vi "ArduinoSerial.vi"() -> ()   [LabVIEW 2014]
uses:
  <vilib>/Instr/_visa.llb/VISA Configure Serial Port (Instr).vi
panel:
  out "XY Graph":cluster{dbl[], dbl[]}(graph)
  out "Y":dbl
  out "X":dbl
  in  "VISA resource name":refnum<visa-resource-name>="COM3"
  in  "baud rate (9600)":u32=9600
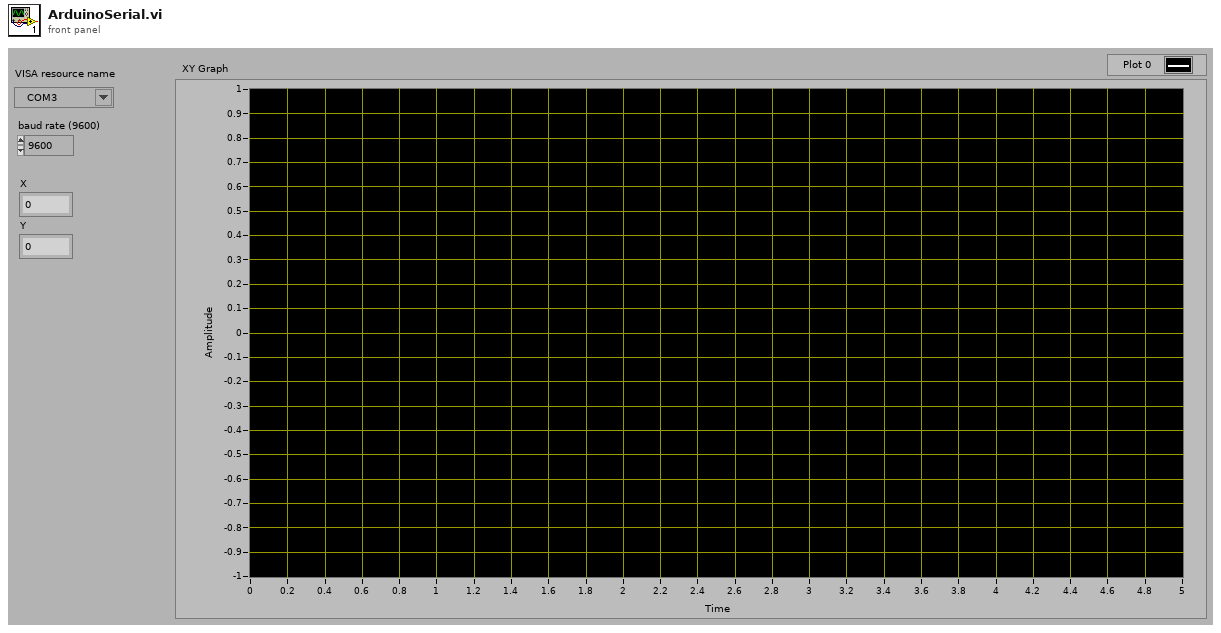
[diagram p1: front panel]
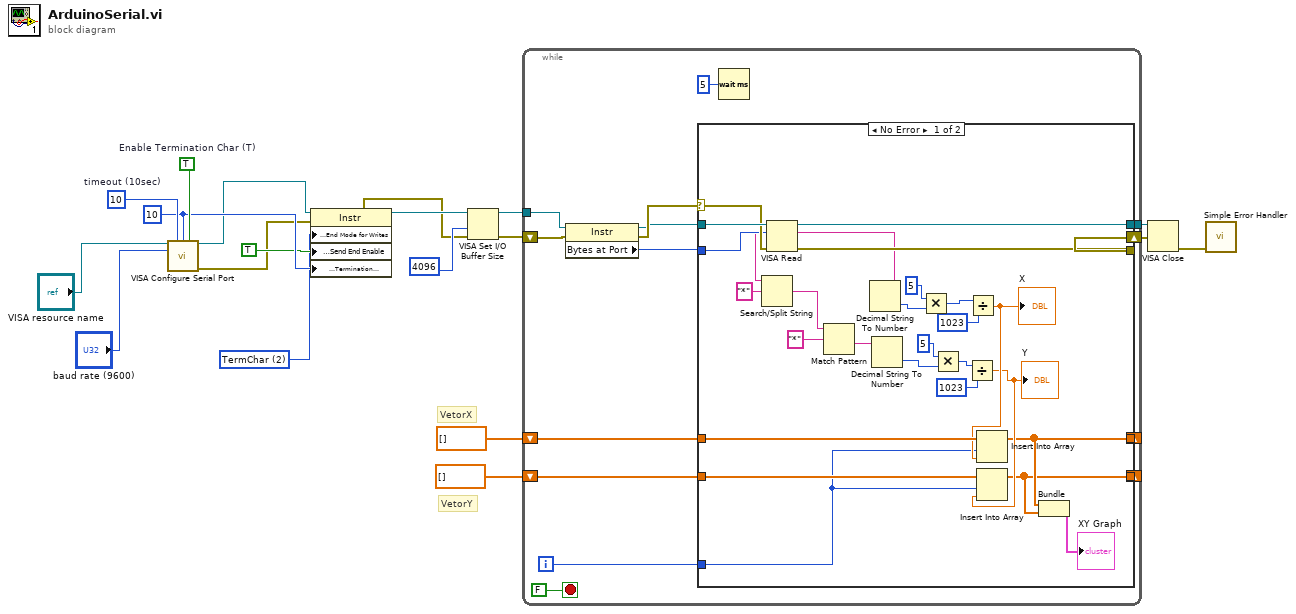
[diagram p0: block diagram]
diagram:
  w12 = u16 2 items=["None", "Last Bit", "TermChar", "Break"] ("Serial Settings:End Mode for Writes")
  w14 = u8 10 ("termination char\n(0xA = '\\n' = LF)")
  w16 = TRUE  # Enable Termination Char (T)
  w17 = u32 10  # timeout (10sec)
  # "VetorY"
  # "VetorX"
  n1 = call-poly "VISA Configure Serial Port"("VISA resource name"="VISA resource name", "timeout (10sec)"=w17, "termination char\n(0xA = '\\n' = LF)"=w14, "Enable Termination\nChar (T)"=w16, "baud rate (9600)"="baud rate (9600)") -> ("VISA resource name out"=w9:refnum<visa-resource-name>, "error out"=w7:errorcluster)  [unwired: 9 in]
  n2 = property class="Instr"(reference=w9, error in=w7, "Serial Settings:End Mode for Writes"=w12, "Message Based Settings:Send End Enable"=TRUE, "Message Based Settings:Termination Character"=w14) -> (reference out=w11:refnum<visa-resource-name>, error out=w10:errorcluster)
  n3 = VISA Set I/O Buffer Size(VISA resource name=w11, size (4096)=u32 4096, error in (no error)=w10) -> (VISA resource name out=w4:refnum<visa-resource-name>, error out=w3:errorcluster)  [unwired: 1 in]
  n4 = while {
    shift-right: [w25] -> w19
    shift-left: w3 -> [w31]
    tunnel: [w27] -> w8
    tunnel: w4 -> [w26]
    shift-right: [w23] -> _
    shift-left: dbl[] [] -> [w24]
    shift-right: [w21] -> _
    shift-left: dbl[] [] -> [w22]
    i -> [w20]
    stop <- FALSE stop-if-true
    n5 = property class="Instr"(reference=w26, error in=w31) -> (reference out=w29:refnum<visa-resource-name>, error out=w30:errorcluster, "Bytes at Port"=w28:u32)
    n6 = case shown="No Error" w30 {
      selector: w30 -> [w58 w62]
      tunnel: w29 -> [w59 w63]
      tunnel: w28 -> [w55 _]
      tunnel: [w57 w63] -> w27
      tunnel: [w56 w62] -> w25
      tunnel: w24 -> [w41 w61]
      tunnel: [w36 w61] -> w23
      tunnel: w22 -> [w39 w60]
      tunnel: [w35 w60] -> w21
      tunnel: w20 -> [w38 _]
      frame No Error {
        n7 = VISA Read(VISA resource name=w59, byte count=w55, error in (no error)=w58) -> (VISA resource name out=w57:refnum<visa-resource-name>, read buffer=w51:string, error out=w56:errorcluster)  [unwired: 1 out]
        n8 = Search/Split String(string=w51, search string/char (-)="*") -> (match + rest of string=w53:string)  [unwired: 1 in, 2 out]
        n9 = Match Pattern(string=w53, regular expression="*" ("search string/char (-)")) -> (after substring=w50:string)  [unwired: 1 in, 3 out]
        n10 = Decimal String To Number(string=w51) -> (number=w49:i32)  [unwired: 2 in, 1 out]
        n11 = Decimal String To Number(string=w50) -> (number=w46:i32)  [unwired: 2 in, 1 out]
        n12 = Multiply(x=5, y=w49) -> (x*y=w45:i32)
        n13 = Multiply(x=5, y=w46) -> (x*y=w42:i32)
        n14 = Divide(x=w42, y=1023) -> (x/y=w37:dbl)
        "Y" <- w37
        n15 = Divide(x=w45, y=1023) -> (x/y=w40:dbl)
        "X" <- w40
        n16 = Insert Into Array(array=w41, index=w38, new element=w40) -> (w36:dbl[])
        n17 = Insert Into Array(array=w39, index=w38, new element=w37) -> (w35:dbl[])
        n18 = Bundle(w36, w35) -> (→"XY Graph":cluster{dbl[], dbl[]})  [unwired: 1 in]
      }
      frame Error {
      }
    }
    n19 = Wait (ms)(milliseconds to wait=u32 5) -> ()  [unwired: 1 out]
  }
  n20 = VISA Close(VISA resource name=w8, error in (no error)=w19) -> (error out=w18:errorcluster)
  n21 = call <vilib>:"Simple Error Handler.vi"("error in (no error)"=w18) -> ()  [unwired: 1 in, 8 out]
